vi "Pre-Build VI - Run Unit Tests.vi"(8 "error in (no error)":errorcluster, 11 "Fail on #todo items":bool) -> (0 "error out":errorcluster, 6 "VIs with #todo bookmarks":string[](array[string]))   [LabVIEW 2021]
uses:
  <vilib>/Utility/miscctls.llb/LVBookmarkInfoTypeDef.ctl
  <vilib>/addons/_JKI Toolkits/Caraya/run-tests/Run Test (Scalar Path).vi
  <vilib>/addons/_JKI Toolkits/Caraya/Caraya.lvlib
panel:
  out "unreadable VIs (errors)":path[](array[path])
  out "VIs with #todo's":map{path, T1}(c390)
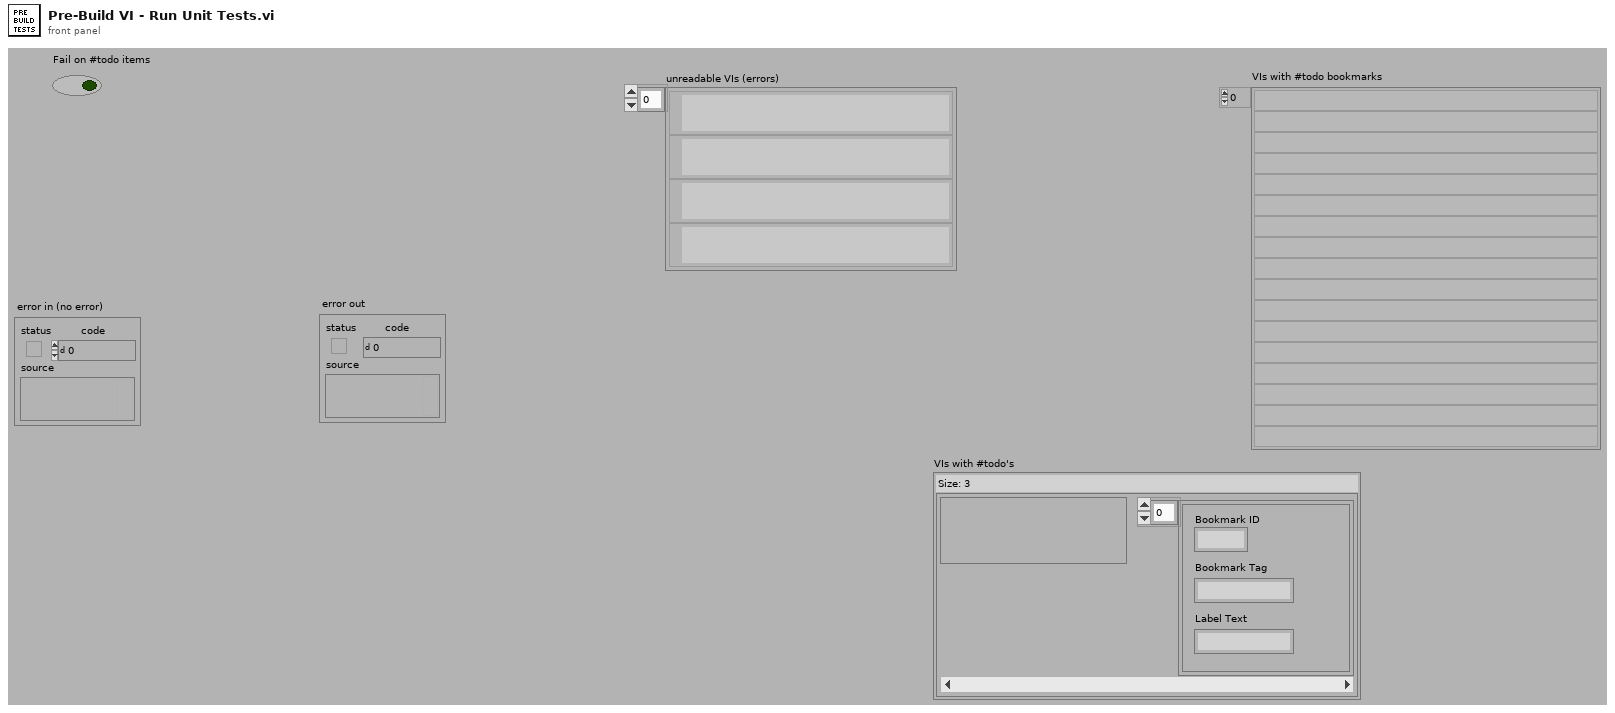
[diagram p1: front panel]
types:
  T1 = typedef "LVBookmarkInfoTypeDef.ctl" = cluster{"Bookmark ID":u32, "Bookmark Tag":string, "Label Text":string}[]
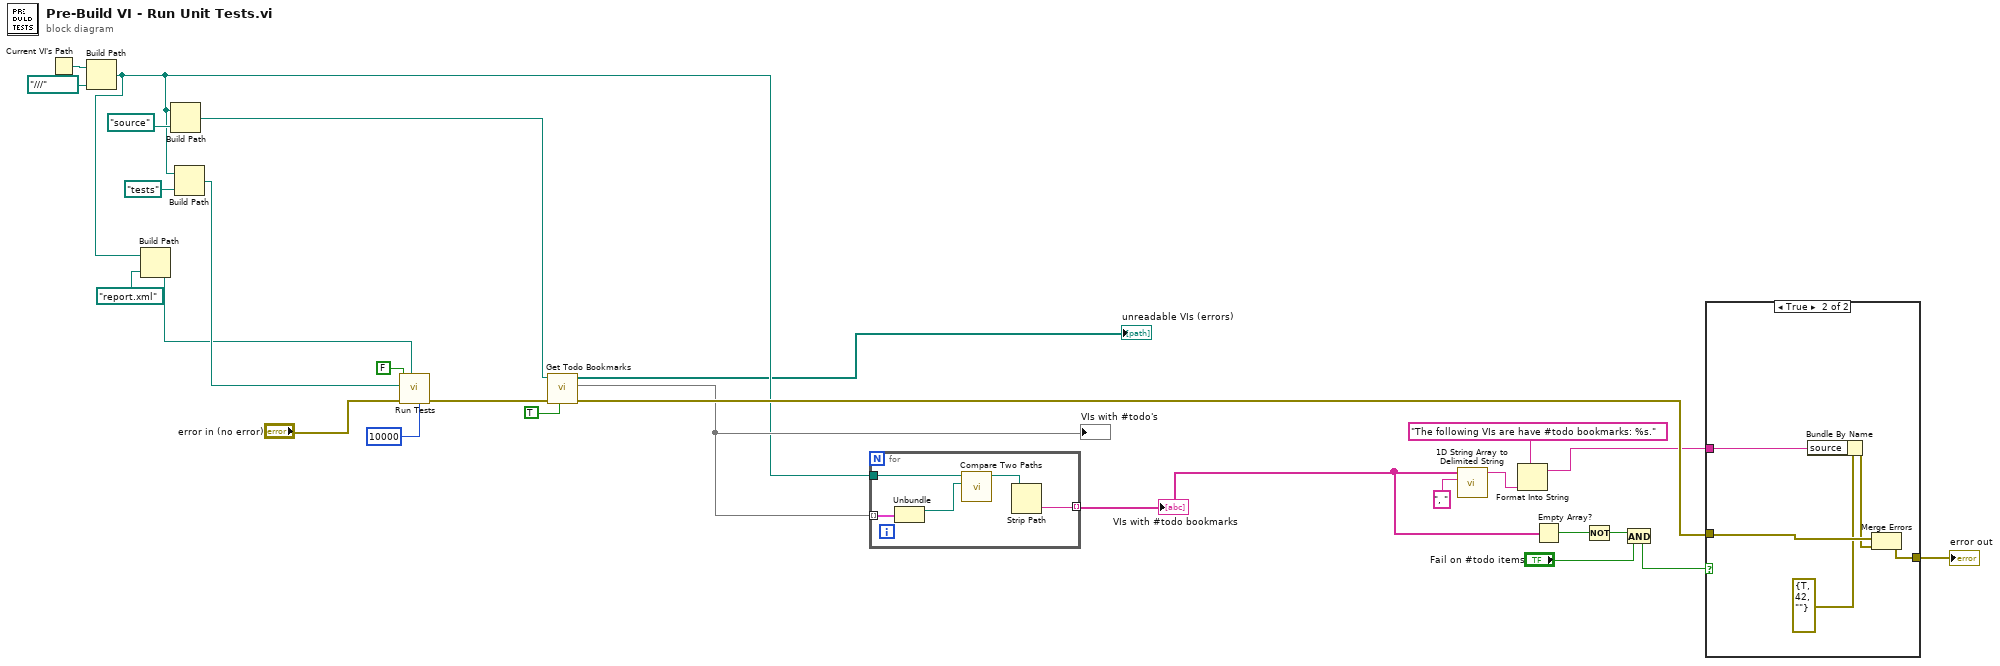
[diagram p0: block diagram]
diagram:
  n1 = Current VI's Path() -> (path=w27:path)
  n2 = Build Path(base path=w27, name or relative path=path "../../../..") -> (appended path=w3:path)
  n3 = Build Path(base path=w3, name or relative path=path "report.xml" ("Relative path (.)")) -> (appended path=w8:path)
  n4 = Build Path(base path=w3, name or relative path=path "source" ("Relative path (.)")) -> (appended path=w23:path)
  n5 = Build Path(base path=w3, name or relative path=path "tests" ("Relative path (.)")) -> (appended path=w11:path)
  n6 = call-poly <vilib>:"Run Tests.vi"("timeout (2000 ms)"=10000, "Report Path"=w8, "error in"="error in (no error)", "Test Path"=w11, "Interactive (T)"=FALSE) -> ("error out"=w5:errorcluster)  [unwired: 5 in, 1 out]
  n7 = call "Get Todo Bookmarks.vi"("open VI references? (False)"=TRUE, "error in (no error)"=w5, "Directory to Search"=w23) -> ("error out"=w22:errorcluster, "todo bookmarks"=w15:map{path, T1}, "unreadable VIs (errors)"=→"unreadable VIs (errors)":path[])  [unwired: 6 in]
  "VIs with #todo's" <- w15
  n8 = for {
    tunnel: w15 -> [w32] mode=indexing
    tunnel: w3 -> [w30]
    tunnel: [w28] -> w17 mode=indexing
    n9 = Unbundle(w32) -> ("key type"=w31:path)  [unwired: 1 out]
    n10 = call <vilib>:"Compare Two Paths.vi"("Path 2"=w31, "Path 1"=w30) -> ("Relative Path from 1 to 2"=w29:path)  [unwired: 6 in, 3 out]
    n11 = Strip Path(path=w29) -> (name=w28:string)  [unwired: 1 out]
  }
  "VIs with #todo bookmarks" <- w17
  n12 = call <vilib>:"1D String Array to Delimited String.vi"("delimiter"=", " ("delimiter (Tab)"), "string array"=w17) -> ("delimited string"=w20:string)  [unwired: 9 in]
  n13 = Format Into String(format string="The following VIs are have #todo bookmarks: %s.", w20) -> (resulting string=w18:string)  [unwired: 2 in, 1 out]
  n14 = Empty Array?(array=w17) -> (empty?=w16:bool)
  n15 = Not(x=w16) -> (.not. x?=w14:bool)
  n16 = And(x=w14, y="Fail on #todo items") -> (x .and. y?=w13:bool)
  n17 = case shown="True" w13 {
    tunnel: w22 -> [w33 w38]
    tunnel: [w33 w34] -> w4
    tunnel: w18 -> [_ w35]
    frame False {
    }
    frame True {
      n18 = Bundle By Name(cluster=errorcluster {"status"=TRUE, "code"=42, "source"=""} ("error out"), "source"=w35) -> (w37:errorcluster)
      n19 = Merge Errors(w38, w37) -> (w34:errorcluster)
    }
  }
  "error out" <- w4
